vi "Launch Async Loop.vi"(8 "error in (no error)":errorcluster, 11 "LoggingControl in":refnum<class "LoggingControl.lvclass">) -> (0 "error out":errorcluster, 3 "LoggingControl out":refnum<class "LoggingControl.lvclass">)   [LabVIEW 2020, in "VolatusGUIElements.lvlib" / "LoggingControl.lvclass"]
uses:
  LoggingControl.lvclass
  LoggingControl.lvclass/LoggingControl.ctl
  Loop Async.vi
  lv-exec-anchor/ExecAnchor/ExecAnchor.lvclass
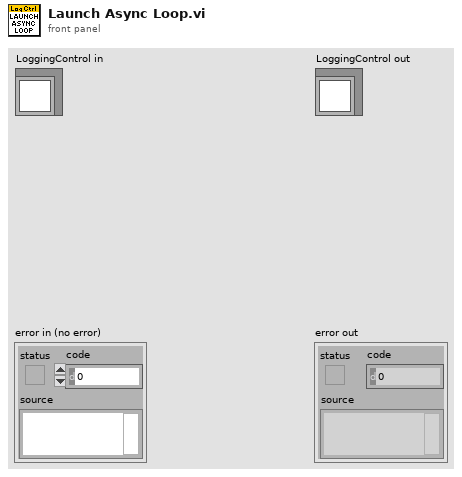
[diagram p1: front panel]
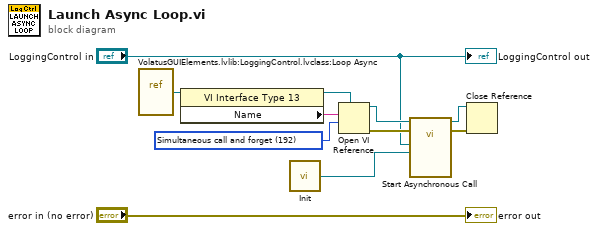
[diagram p0: block diagram]
diagram:
  w5 = 192 items=["Record modifications"=1, "Open templates for editing"=2, "Prompt user to save"=4, "Prepare for reentrant run"=8, "Prompt to find missing subVIs"=16, "Hide loading dialog box"=32, "Enable simultaneous calls"=64, "Prepare to call and forget"=128, "Simultaneous call and forget"=192, "Prepare to call and collect"=256, "Simultaneous call and collect"=320]
  n1 = vi-ref "VolatusGUIElements.lvlib:LoggingControl.lvclass:Loop Async.vi"() -> (w3:refnum<vi>)
  n2 = property class="VI Interface Type 13"(reference=w3) -> (reference out=w6:refnum<vi>, "Name"=w4:string)  [unwired: 1 in, 1 out]
  n3 = call "Init.vi"() -> ("ExecAnchor out"=w1:refnum<class "ExecAnchor.lvclass">)  [unwired: 7 in]
  n4 = Open VI Reference(type specifier VI Refnum (for type only)=w6, vi path=w4, options=w5) -> (vi reference=w8:refnum<vi>, error out=w7:errorcluster)  [unwired: 3 in]
  n5 = call-by-ref "Start Asynchronous Call"(reference=w8, error in=w7, "ExecAnchor"=w1, "LoggingControl in"="LoggingControl in") -> (reference out=w10:refnum<vi>, error out=w9:errorcluster)  [unwired: 9 in, 1 out]
  n6 = Close Reference(reference=w10, error in (no error)=w9) -> ()  [unwired: 1 out]
  "error out" <- "error in (no error)"
  "LoggingControl out" <- "LoggingControl in"
